vi "Set boolean controls value.vi"(9 "Value":bool, 11 "Boolean ctrl ref array":refnum<vi>[](array[refnum])) -> ()   [LabVIEW 2017]
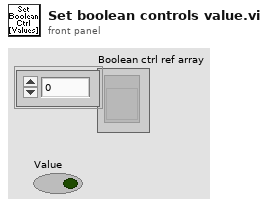
[diagram p1: front panel]
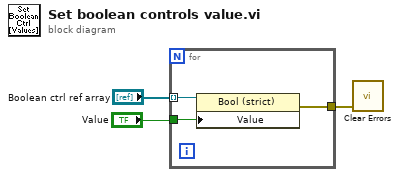
[diagram p0: block diagram]
diagram:
  n1 = for {
    tunnel: "Boolean ctrl ref array" -> [w6] mode=indexing
    tunnel: "Value" -> [w5]
    tunnel: [w4] -> w1
    n2 = property on="Property Node" class="Bool (strict)"(reference=w6, "Value"=w5) -> (error out=w4:errorcluster)  [unwired: 1 in, 1 out]
  }
  n3 = call <vilib>:"Clear Errors.vi"("error in (no error)"=w1) -> ()  [unwired: 5 in, 2 out]
